vi "Comm String Send CMD.vi"(0 "niDTS Comm Serial in":refnum<class "niDTS Comm Serial.lvclass">, 5 "Command":string, 11 "error in (no error)":errorcluster) -> (4 "niDTS Comm Serial out":refnum<class "niDTS Comm Serial.lvclass">, 15 "error out":errorcluster)   [LabVIEW 2015, in "niDTS CommLib.lvlib" / "niDTS Comm Serial.lvclass"]
uses:
  niDTS Comm Serial.lvclass
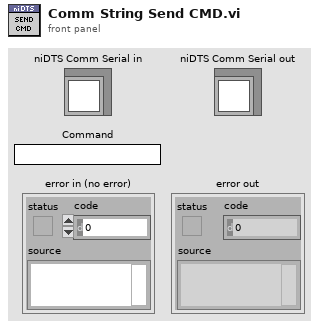
[diagram p1: front panel]
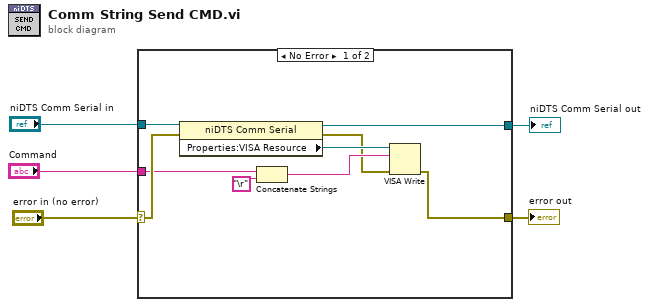
[diagram p0: block diagram]
diagram:
  n1 = case shown="No Error" "error in (no error)" {
    selector: "error in (no error)" -> [w13 w16]
    tunnel: "Command" -> [w11 _]
    tunnel: "niDTS Comm Serial in" -> [w14 w15]
    tunnel: [w7 w16] -> w2
    tunnel: [w6 w15] -> w1
    frame No Error {
      n2 = property class="niDTS Comm Serial"(reference=w14, error in=w13) -> (reference out=w6:refnum<class "niDTS Comm Serial.lvclass">, error out=w8:errorcluster, "Properties:VISA Resource"=w10:refnum<visa-resource-name>)
      n3 = Concatenate Strings(w11, "\r") -> (w9:string)
      n4 = VISA Write(VISA resource name=w10, write buffer=w9, error in (no error)=w8) -> (error out=w7:errorcluster)  [unwired: 2 out]
    }
    frame Error {
    }
  }
  "error out" <- w2
  "niDTS Comm Serial out" <- w1
